vi "Get Session Elapsed Time.vi"(6 "timeout (ms)":i32=-1, 8 "error in (no error)":errorcluster, 11 "FlexLogger_gRPCAPI in":refnum<class "FlexLogger_gRPC.lvclass">) -> (0 "error out":errorcluster, 2 "Elapsed Time":i32, 3 "FlexLogger_gRPCAPI out":refnum<class "FlexLogger_gRPC.lvclass">)   [LabVIEW 2020, in "FlexLogger_gRPC.lvlib" / "FlexLogger_gRPC.lvclass"]
uses:
  FlexLogger_gRPC.lvclass
  FlexLogger_gRPC.lvclass/FlexLogger_gRPC.ctl
  FlexLogger_client/FlexLogger_client.lvlib
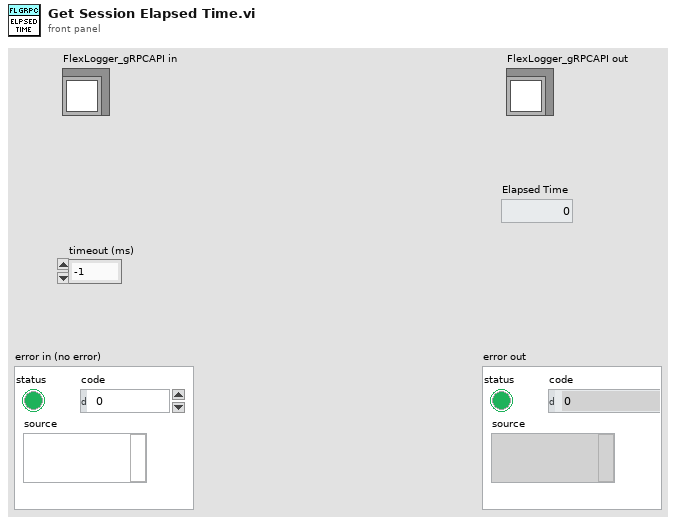
[diagram p1: front panel]
types:
  T1 = typedef "grpc-lvsupport-release.lvlib/grpcId.ctl" = u64
  T2 = typedef "FlexLogger_client.lvlib/flexlogger_GetElapsedTestTimeResponse.ctl" = cluster{"elapsed_test_time":dbl}
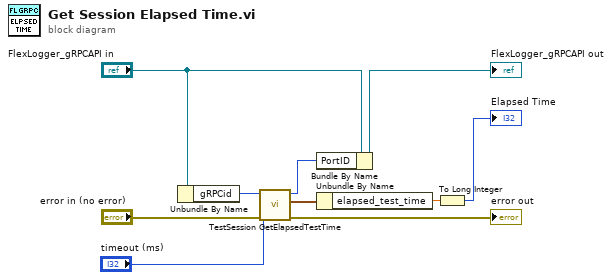
[diagram p0: block diagram]
diagram:
  n1 = Unbundle By Name("FlexLogger_gRPCAPI in") -> ("gRPCid"=w6:T1)
  n2 = call "TestSession GetElapsedTestTime.vi"("error in"="error in (no error)", "timeout (ms)"="timeout (ms)", "gRPC ID"=w6) -> ("error out"=→"error out":errorcluster, "Response Data"=w10:T2, "gRPC ID out"=w3:T1)  [unwired: 6 in]
  n3 = Bundle By Name(cluster="FlexLogger_gRPCAPI in", "PortID"=w3) -> (→"FlexLogger_gRPCAPI out":refnum<class "FlexLogger_gRPC.lvclass">)
  n4 = Unbundle By Name(w10) -> ("elapsed_test_time"=w9:dbl)
  n5 = To Long Integer(number=w9) -> (32bit integer=→"Elapsed Time":i32)
